vi "Write E5071C_VISA.vi"(8 "error in (no error)":errorcluster, 10 "E5071C_VISA":refnum<visa-resource-name>, 11 "E5071C in":refnum<class "E5071C.lvclass">) -> (0 "error out":errorcluster, 3 "E5071C out":refnum<class "E5071C.lvclass">)   [LabVIEW 2020, in "E5071C.lvlib" / "E5071C.lvclass"]
uses:
  E5071C.lvclass
  E5071C.lvclass/E5071C.ctl
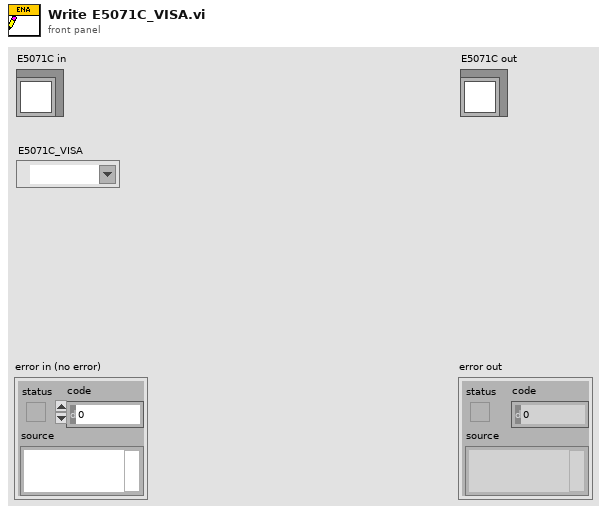
[diagram p1: front panel]
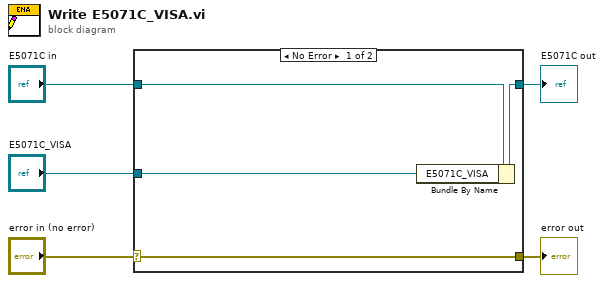
[diagram p0: block diagram]
diagram:
  n1 = case shown="No Error" "error in (no error)" {
    selector: "error in (no error)" -> [w9 w10]
    tunnel: [w9 w10] -> w4
    tunnel: [w7 w11] -> w2
    tunnel: "E5071C in" -> [w8 w11]
    tunnel: "E5071C_VISA" -> [w6 _]
    frame No Error {
      n2 = Bundle By Name(cluster=w8, "E5071C_VISA"=w6) -> (w7:refnum<class "E5071C.lvclass">)
    }
    frame Error {
    }
  }
  "error out" <- w4
  "E5071C out" <- w2
